vi "laser-shutter-control-subvi.vi"(7 "Camera Shutter":bool, 8 "error in":errorcluster, 9 "VISA resource name out":refnum<visa-resource-name>, 10 "Wheel Speed":u8, 11 "Laser Shutter":T1) -> (0 "error out":errorcluster, 1 "Status":bool, 3 "Current Filterwheel":string)   [LabVIEW 2014]
uses:
  ctts/laser shutters.ctl
  Global Shutter Variables - SubVI.vi
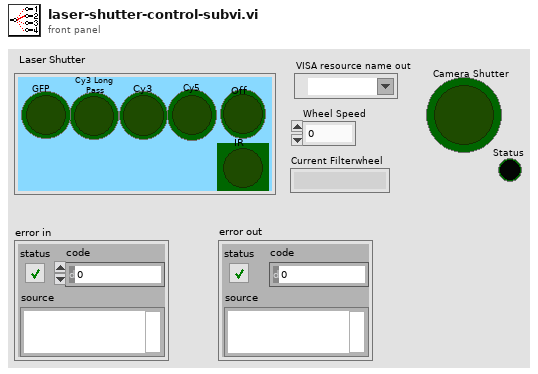
[diagram p1: front panel]
types:
  T1 = typedef "laser shutters.ctl" = enum32{"No Selection", "GFP", "Cy3 Long \nPass", "Cy3", "Cy5", "Off", "IR"}
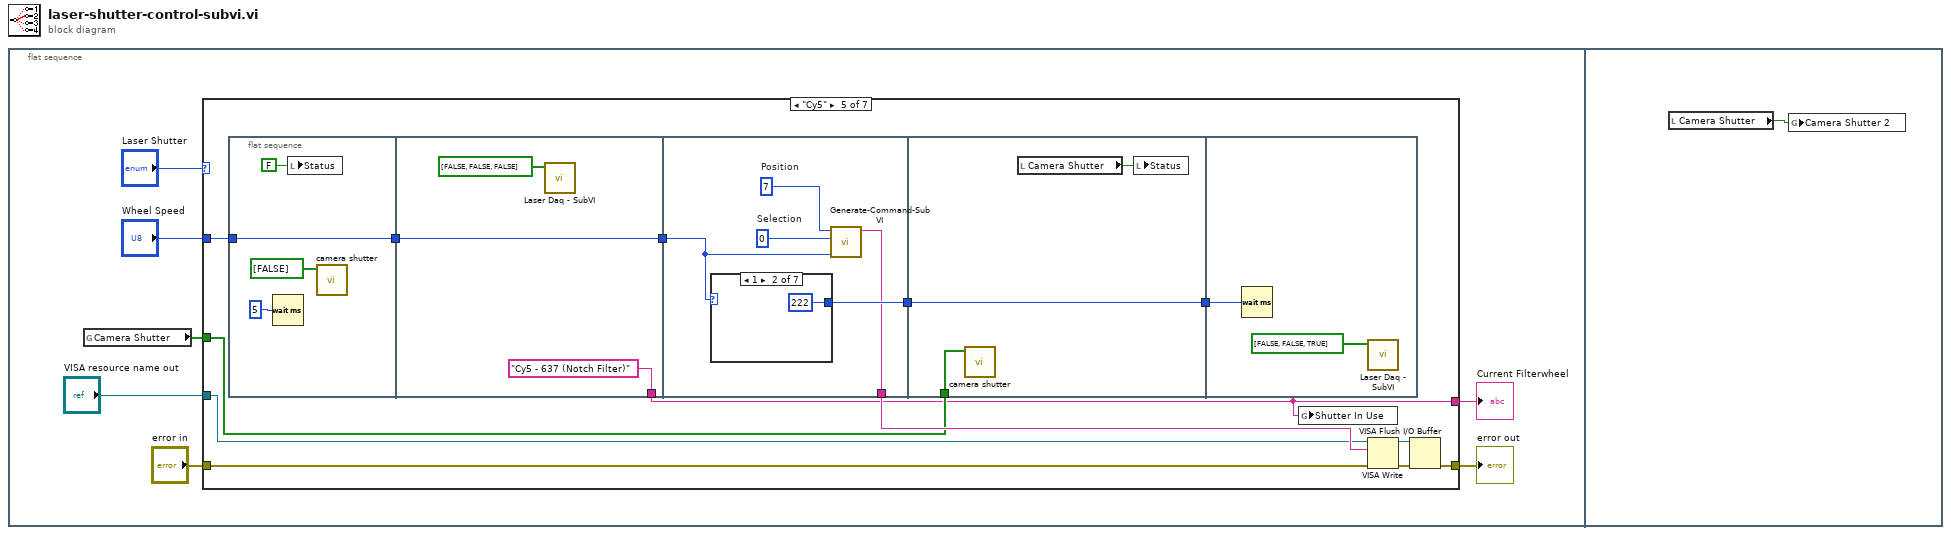
[diagram p0: block diagram]
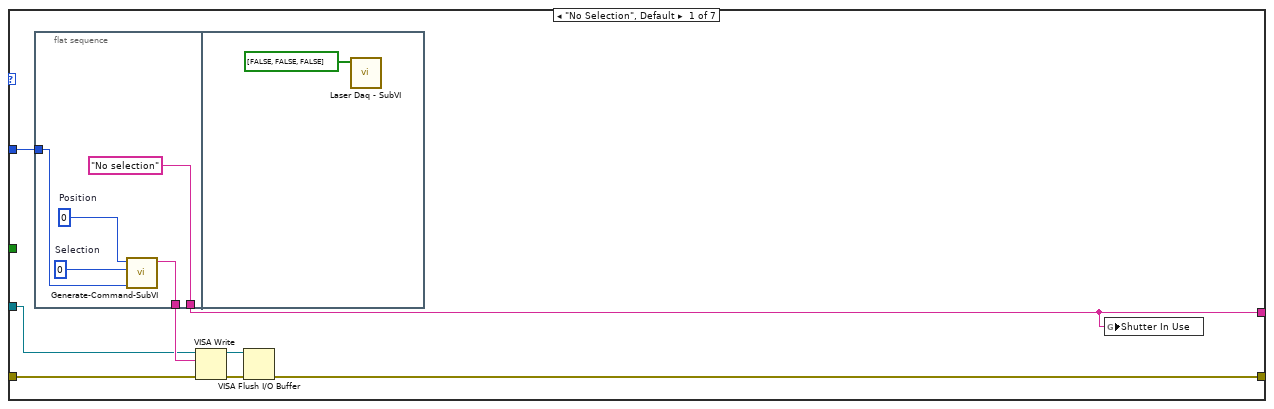
[diagram p2: hidden frame]
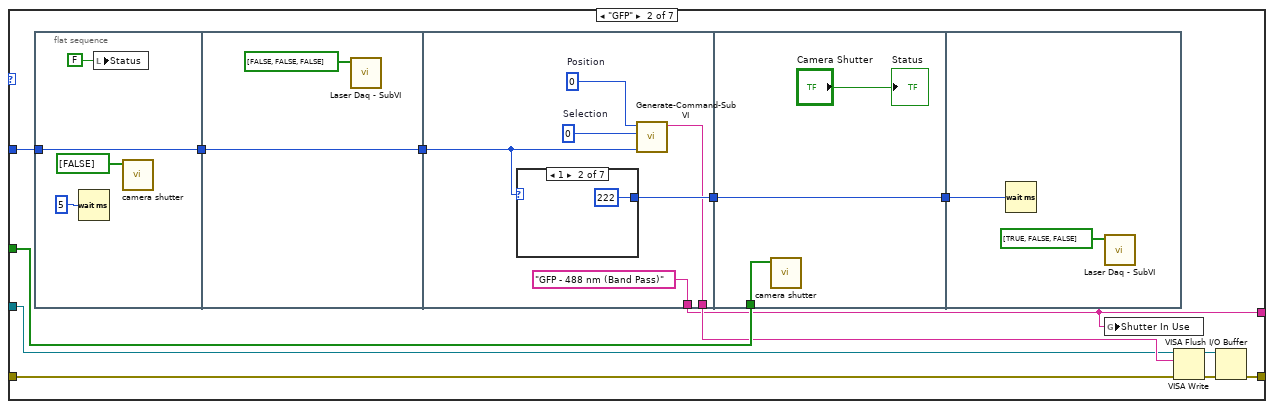
[diagram p3: hidden frame]
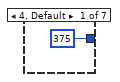
[diagram p4: hidden frame]
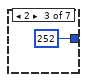
[diagram p5: hidden frame]
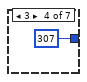
[diagram p6: hidden frame]
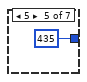
[diagram p7: hidden frame]
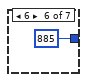
[diagram p8: hidden frame]
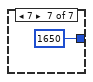
[diagram p9: hidden frame]
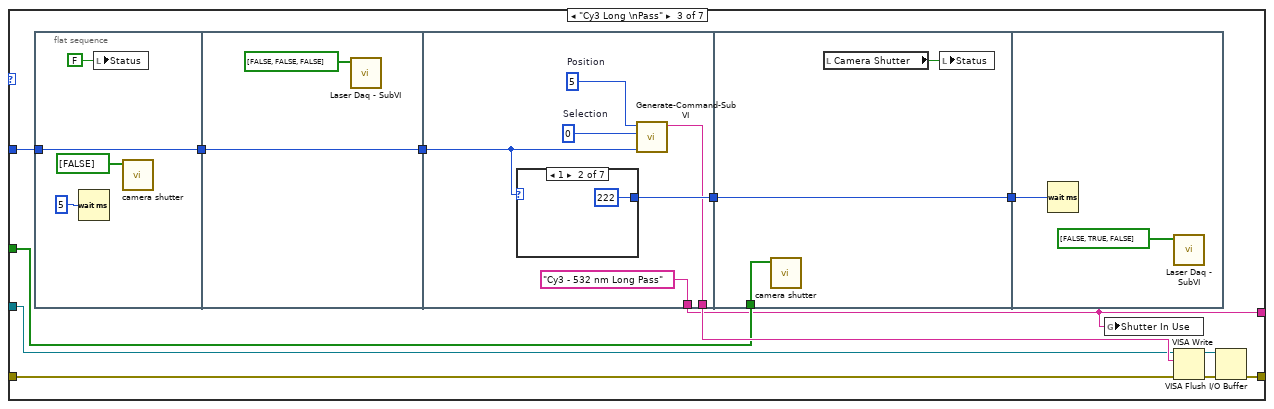
[diagram p10: hidden frame]
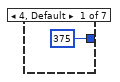
[diagram p11: hidden frame]
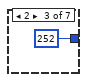
[diagram p12: hidden frame]
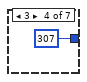
[diagram p13: hidden frame]
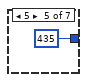
[diagram p14: hidden frame]
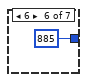
[diagram p15: hidden frame]
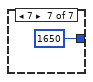
[diagram p16: hidden frame]
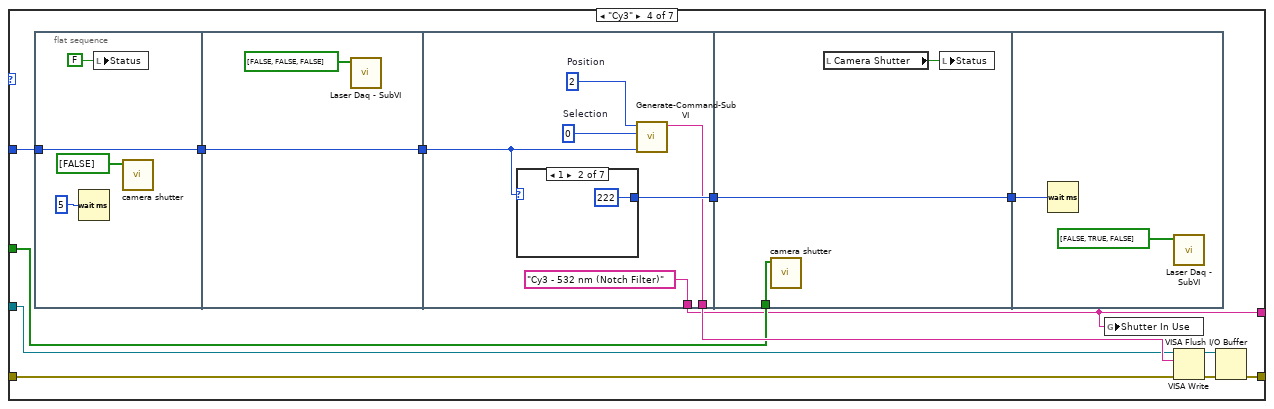
[diagram p17: hidden frame]
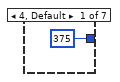
[diagram p18: hidden frame]
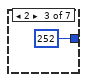
[diagram p19: hidden frame]
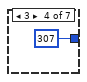
[diagram p20: hidden frame]
diagram:
  n1 = flat-sequence {
    frame #0 {
      n2 = global read "Global Shutter Variables - SubVI.vi" "Camera Shutter"() -> (w5:bool[])
      n3 = case shown="\"Cy5\"" "Laser Shutter" {
        tunnel: "Wheel Speed" -> [w14 w33 w63 w97 w137 _ w188]
        tunnel: w5 -> [_ w31 w62 w99 w135 w172 _]
        tunnel: "VISA resource name out" -> [w10 w27 w64 w101 w138 _ w185]
        tunnel: "error in" -> [w9 w26 w61 w100 w136 w170 w184]
        tunnel: [w8 w23 w60 w98 w134 w170 w182] -> w1
        tunnel: [w15 w22 w59 w96 w133 w171 w183] -> w2
        frame "No Selection", Default {
          n4 = flat-sequence {
            tunnel: ["No selection"] -> w15
            tunnel: w14 -> [w17]
            tunnel: [w16] -> w11
            frame #0 {
              w18 = 0  # Selection
              w19 = 0  # Position
              n5 = call "Generate-Command-SubVI.vi"("Wheel Speed"=w17, "Wheel Selection"=w18, "Wheel Position"=w19) -> ("type"=w16:string)  [unwired: 8 in]
            }
            frame #1 {
              n6 = call "Laser Daq - SubVI.vi"("Array"=bool[] [FALSE, FALSE, FALSE]) -> ()  [unwired: 11 in]
            }
          }
          n7 = VISA Write(VISA resource name=w10, write buffer=w11, error in (no error)=w9) -> (VISA resource name out=w12:refnum<visa-resource-name>, error out=w13:errorcluster)  [unwired: 1 out]
          n8 = VISA Flush I/O Buffer(VISA resource name=w12, error in (no error)=w13) -> (error out=w8:errorcluster)  [unwired: 1 in, 1 out]
          n9 = global write "Global Shutter Variables - SubVI.vi" "Shutter In Use"(w15) -> ()
        }
        frame "GFP" {
          n10 = flat-sequence {
            tunnel: [w35] -> w34
            tunnel: w33 -> [w35]
            tunnel: w34 -> [w39]
            tunnel: [w39] -> w32
            tunnel: w32 -> [w44]
            tunnel: [w43] -> w30
            tunnel: [w42] -> w28
            tunnel: ["GFP - 488 nm (Band Pass)"] -> w22
            tunnel: w31 -> [w56]
            tunnel: w30 -> [w55]
            tunnel: [w55] -> w29
            tunnel: w29 -> [w57]
            frame #0 {
              n11 = Wait (ms)(milliseconds to wait=5) -> ()  [unwired: 1 out]
              n12 = local write "Status"(FALSE) -> ()
              n13 = call "camera shutter.vi"("Camera Input Switch"=bool[] [FALSE]) -> ()  [unwired: 10 in, 1 out]
            }
            frame #1 {
              n14 = call "Laser Daq - SubVI.vi"("Array"=bool[] [FALSE, FALSE, FALSE]) -> ()  [unwired: 11 in]
            }
            frame #2 {
              w45 = 0  # Selection
              w46 = 0  # Position
              n15 = case shown="1" w44 {
                tunnel: [375 222 252 307 435 885 1650] -> w43
                frame 4, Default {
                }
                frame 1 {
                }
                frame 2 {
                }
                frame 3 {
                }
                frame 5 {
                }
                frame 6 {
                }
                frame 7 {
                }
              }
              n16 = call "Generate-Command-SubVI.vi"("Wheel Speed"=w44, "Wheel Selection"=w45, "Wheel Position"=w46) -> ("type"=w42:string)  [unwired: 8 in]
            }
            frame #3 {
              n17 = call "camera shutter.vi"("Camera Input Switch"=w56) -> ()  [unwired: 10 in, 1 out]
              "Status" <- "Camera Shutter"
            }
            frame #4 {
              n18 = Wait (ms)(milliseconds to wait=w57) -> ()  [unwired: 1 out]
              n19 = call "Laser Daq - SubVI.vi"("Array"=bool[] [TRUE, FALSE, FALSE]) -> ()  [unwired: 11 in]
            }
          }
          n20 = global write "Global Shutter Variables - SubVI.vi" "Shutter In Use"(w22) -> ()
          n21 = VISA Write(VISA resource name=w27, write buffer=w28, error in (no error)=w26) -> (VISA resource name out=w25:refnum<visa-resource-name>, error out=w24:errorcluster)  [unwired: 1 out]
          n22 = VISA Flush I/O Buffer(VISA resource name=w25, error in (no error)=w24) -> (error out=w23:errorcluster)  [unwired: 1 in, 1 out]
        }
        frame "Cy3 Long \nPass" {
          n23 = flat-sequence {
            tunnel: [w72] -> w71
            tunnel: w63 -> [w72]
            tunnel: w71 -> [w76]
            tunnel: [w76] -> w70
            tunnel: w70 -> [w81]
            tunnel: [w80] -> w69
            tunnel: [w79] -> w67
            tunnel: ["Cy3 - 532 nm Long Pass"] -> w59
            tunnel: w62 -> [w93]
            tunnel: w69 -> [w91]
            tunnel: [w91] -> w68
            tunnel: w68 -> [w94]
            frame #0 {
              n24 = Wait (ms)(milliseconds to wait=5) -> ()  [unwired: 1 out]
              n25 = local write "Status"(FALSE) -> ()
              n26 = call "camera shutter.vi"("Camera Input Switch"=bool[] [FALSE]) -> ()  [unwired: 10 in, 1 out]
            }
            frame #1 {
              n27 = call "Laser Daq - SubVI.vi"("Array"=bool[] [FALSE, FALSE, FALSE]) -> ()  [unwired: 11 in]
            }
            frame #2 {
              w82 = 0  # Selection
              w83 = 5  # Position
              n28 = case shown="1" w81 {
                tunnel: [375 222 252 307 435 885 1650] -> w80
                frame 4, Default {
                }
                frame 1 {
                }
                frame 2 {
                }
                frame 3 {
                }
                frame 5 {
                }
                frame 6 {
                }
                frame 7 {
                }
              }
              n29 = call "Generate-Command-SubVI.vi"("Wheel Speed"=w81, "Wheel Selection"=w82, "Wheel Position"=w83) -> ("type"=w79:string)  [unwired: 8 in]
            }
            frame #3 {
              n30 = call "camera shutter.vi"("Camera Input Switch"=w93) -> ()  [unwired: 10 in, 1 out]
              n31 = local read "Camera Shutter"() -> (w92:bool)
              n32 = local write "Status"(w92) -> ()
            }
            frame #4 {
              n33 = Wait (ms)(milliseconds to wait=w94) -> ()  [unwired: 1 out]
              n34 = call "Laser Daq - SubVI.vi"("Array"=bool[] [FALSE, TRUE, FALSE]) -> ()  [unwired: 11 in]
            }
          }
          n35 = global write "Global Shutter Variables - SubVI.vi" "Shutter In Use"(w59) -> ()
          n36 = VISA Write(VISA resource name=w64, write buffer=w67, error in (no error)=w61) -> (VISA resource name out=w66:refnum<visa-resource-name>, error out=w65:errorcluster)  [unwired: 1 out]
          n37 = VISA Flush I/O Buffer(VISA resource name=w66, error in (no error)=w65) -> (error out=w60:errorcluster)  [unwired: 1 in, 1 out]
        }
        frame "Cy3" {
          n38 = flat-sequence {
            tunnel: [w109] -> w108
            tunnel: w97 -> [w109]
            tunnel: w108 -> [w113]
            tunnel: [w113] -> w107
            tunnel: w107 -> [w118]
            tunnel: [w117] -> w106
            tunnel: [w116] -> w104
            tunnel: ["Cy3 - 532 nm (Notch Filter)"] -> w96
            tunnel: w99 -> [w130]
            tunnel: w106 -> [w128]
            tunnel: [w128] -> w105
            tunnel: w105 -> [w131]
            frame #0 {
              n39 = Wait (ms)(milliseconds to wait=5) -> ()  [unwired: 1 out]
              n40 = local write "Status"(FALSE) -> ()
              n41 = call "camera shutter.vi"("Camera Input Switch"=bool[] [FALSE]) -> ()  [unwired: 10 in, 1 out]
            }
            frame #1 {
              n42 = call "Laser Daq - SubVI.vi"("Array"=bool[] [FALSE, FALSE, FALSE]) -> ()  [unwired: 11 in]
            }
            frame #2 {
              w119 = 0  # Selection
              w120 = 2  # Position
              n43 = case shown="1" w118 {
                tunnel: [375 222 252 307 435 885 1650] -> w117
                frame 4, Default {
                }
                frame 1 {
                }
                frame 2 {
                }
                frame 3 {
                }
                frame 5 {
                }
                frame 6 {
                }
                frame 7 {
                }
              }
              n44 = call "Generate-Command-SubVI.vi"("Wheel Speed"=w118, "Wheel Selection"=w119, "Wheel Position"=w120) -> ("type"=w116:string)  [unwired: 8 in]
            }
            frame #3 {
              n45 = call "camera shutter.vi"("Camera Input Switch"=w130) -> ()  [unwired: 10 in, 1 out]
              n46 = local read "Camera Shutter"() -> (w129:bool)
              n47 = local write "Status"(w129) -> ()
            }
            frame #4 {
              n48 = Wait (ms)(milliseconds to wait=w131) -> ()  [unwired: 1 out]
              n49 = call "Laser Daq - SubVI.vi"("Array"=bool[] [FALSE, TRUE, FALSE]) -> ()  [unwired: 11 in]
            }
          }
          n50 = global write "Global Shutter Variables - SubVI.vi" "Shutter In Use"(w96) -> ()
          n51 = VISA Write(VISA resource name=w101, write buffer=w104, error in (no error)=w100) -> (VISA resource name out=w103:refnum<visa-resource-name>, error out=w102:errorcluster)  [unwired: 1 out]
          n52 = VISA Flush I/O Buffer(VISA resource name=w103, error in (no error)=w102) -> (error out=w98:errorcluster)  [unwired: 1 in, 1 out]
        }
        frame "Cy5" {
          n53 = flat-sequence {
            tunnel: [w146] -> w145
            tunnel: w137 -> [w146]
            tunnel: w145 -> [w151]
            tunnel: [w151] -> w144
            tunnel: ["Cy5 - 637 (Notch Filter)"] -> w133
            tunnel: w144 -> [w155]
            tunnel: [w154] -> w143
            tunnel: [w153] -> w141
            tunnel: w135 -> [w167]
            tunnel: w143 -> [w165]
            tunnel: [w165] -> w142
            tunnel: w142 -> [w168]
            frame #0 {
              n54 = Wait (ms)(milliseconds to wait=5) -> ()  [unwired: 1 out]
              n55 = local write "Status"(FALSE) -> ()
              n56 = call "camera shutter.vi"("Camera Input Switch"=bool[] [FALSE]) -> ()  [unwired: 10 in, 1 out]
            }
            frame #1 {
              n57 = call "Laser Daq - SubVI.vi"("Array"=bool[] [FALSE, FALSE, FALSE]) -> ()  [unwired: 11 in]
            }
            frame #2 {
              w156 = 0  # Selection
              w157 = 7  # Position
              n58 = case shown="1" w155 {
                tunnel: [375 222 252 307 435 885 1650] -> w154
                frame 4, Default {
                }
                frame 1 {
                }
                frame 2 {
                }
                frame 3 {
                }
                frame 5 {
                }
                frame 6 {
                }
                frame 7 {
                }
              }
              n59 = call "Generate-Command-SubVI.vi"("Wheel Speed"=w155, "Wheel Selection"=w156, "Wheel Position"=w157) -> ("type"=w153:string)  [unwired: 8 in]
            }
            frame #3 {
              n60 = call "camera shutter.vi"("Camera Input Switch"=w167) -> ()  [unwired: 10 in, 1 out]
              n61 = local read "Camera Shutter"() -> (w166:bool)
              n62 = local write "Status"(w166) -> ()
            }
            frame #4 {
              n63 = Wait (ms)(milliseconds to wait=w168) -> ()  [unwired: 1 out]
              n64 = call "Laser Daq - SubVI.vi"("Array"=bool[] [FALSE, FALSE, TRUE]) -> ()  [unwired: 11 in]
            }
          }
          n65 = global write "Global Shutter Variables - SubVI.vi" "Shutter In Use"(w133) -> ()
          n66 = VISA Write(VISA resource name=w138, write buffer=w141, error in (no error)=w136) -> (VISA resource name out=w140:refnum<visa-resource-name>, error out=w139:errorcluster)  [unwired: 1 out]
          n67 = VISA Flush I/O Buffer(VISA resource name=w140, error in (no error)=w139) -> (error out=w134:errorcluster)  [unwired: 1 in, 1 out]
        }
        frame "IR" {
          n68 = flat-sequence {
            tunnel: [""] -> w171
            tunnel: w172 -> [w179]
            frame #0 {
              n69 = Wait (ms)(milliseconds to wait=5) -> ()  [unwired: 1 out]
              n70 = local write "Status"(FALSE) -> ()
              n71 = call "camera shutter.vi"("Camera Input Switch"=bool[] [FALSE]) -> ()  [unwired: 10 in, 1 out]
            }
            frame #1 {
              n72 = call "Laser Daq - SubVI.vi"("Array"=bool[] [FALSE, FALSE, FALSE]) -> ()  [unwired: 11 in]
            }
            frame #2 {
            }
            frame #3 {
              n73 = call "camera shutter.vi"("Camera Input Switch"=w179) -> ()  [unwired: 10 in, 1 out]
              n74 = local read "Camera Shutter"() -> (w178:bool)
              n75 = local write "Status"(w178) -> ()
            }
            frame #4 {
              n76 = call "Laser Daq - SubVI.vi"("Array"=bool[] [TRUE, FALSE, FALSE]) -> ()  [unwired: 11 in]
            }
          }
        }
        frame "Off" {
          n77 = flat-sequence {
            tunnel: w188 -> [w191]
            tunnel: ["No filter (blocked)"] -> w183
            tunnel: [w189] -> w181
            frame #0 {
              w192 = 0  # Selection
              w193 = 0  # Position
              n78 = call "Generate-Command-SubVI.vi"("Wheel Speed"=w191, "Wheel Selection"=w192, "Wheel Position"=w193) -> ("type"=w189:string)  [unwired: 8 in]
            }
            frame #1 {
              w195 = bool[] [FALSE]
              w194 = FALSE
              n79 = call "camera shutter.vi"("Camera Input Switch"=w195) -> ()  [unwired: 10 in, 1 out]
              n80 = global write "Global Shutter Variables - SubVI.vi" "Camera Shutter"(w195) -> ()
              n81 = local write "Status"(w194) -> ()
              n82 = local write "Camera Shutter"(w194) -> ()
              n83 = global write "Global Shutter Variables - SubVI.vi" "Camera Shutter 2"(w194) -> ()
            }
            frame #2 {
              n84 = call "Laser Daq - SubVI.vi"("Array"=bool[] [FALSE, FALSE, FALSE]) -> ()  [unwired: 11 in]
            }
          }
          n85 = VISA Write(VISA resource name=w185, write buffer=w181, error in (no error)=w184) -> (VISA resource name out=w186:refnum<visa-resource-name>, error out=w187:errorcluster)  [unwired: 1 out]
          n86 = VISA Flush I/O Buffer(VISA resource name=w186, error in (no error)=w187) -> (error out=w182:errorcluster)  [unwired: 1 in, 1 out]
          n87 = global write "Global Shutter Variables - SubVI.vi" "Shutter In Use"(w183) -> ()
        }
      }
      "Current Filterwheel" <- w2
      "error out" <- w1
    }
    frame #1 {
      n88 = local read "Camera Shutter"() -> (w197:bool)
      n89 = global write "Global Shutter Variables - SubVI.vi" "Camera Shutter 2"(w197) -> ()
    }
  }
